vi "Write Path.vi"(8 "error in (no error)":errorcluster, 10 "Path":path, 11 "TXT_Writer in":refnum<class "TXT_Writer.lvclass">) -> (0 "error out":errorcluster, 3 "TXT_Writer out":refnum<class "TXT_Writer.lvclass">)   [LabVIEW 2024, in "Data.lvlib" / "TXT_Writer.lvclass"]
uses:
  TXT_Writer.lvclass
  TXT_Writer.lvclass/TXT_Writer.ctl
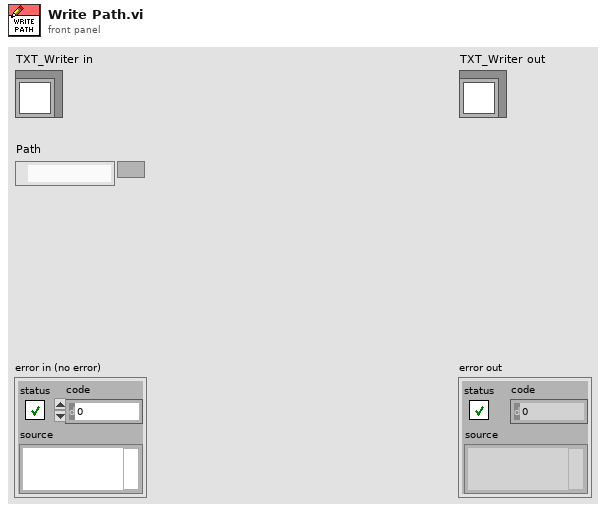
[diagram p1: front panel]
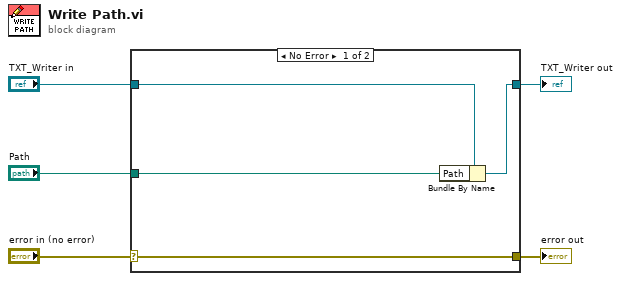
[diagram p0: block diagram]
diagram:
  n1 = case shown="No Error" "error in (no error)" {
    selector: "error in (no error)" -> [w9 w10]
    tunnel: [w9 w10] -> w4
    tunnel: [w7 w11] -> w2
    tunnel: "TXT_Writer in" -> [w8 w11]
    tunnel: "Path" -> [w6 _]
    frame No Error {
      n2 = Bundle By Name(cluster=w8, "Path"=w6) -> (w7:refnum<class "TXT_Writer.lvclass">)
    }
    frame Error {
    }
  }
  "error out" <- w4
  "TXT_Writer out" <- w2
